vi "OpenExcel.vi"(1 "Visible(T)":bool=TRUE, 2 "error in (no error)":errorcluster caption="错误输入（无错误）", 4 "输入Excel路径":path) -> (0 "error out":errorcluster caption="错误输出")   [LabVIEW 2018]
panel:
  in  "Excel._Application":refnum<k7>
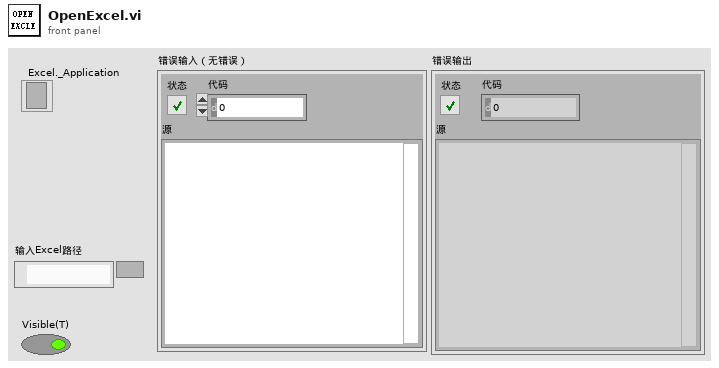
[diagram p1: front panel]
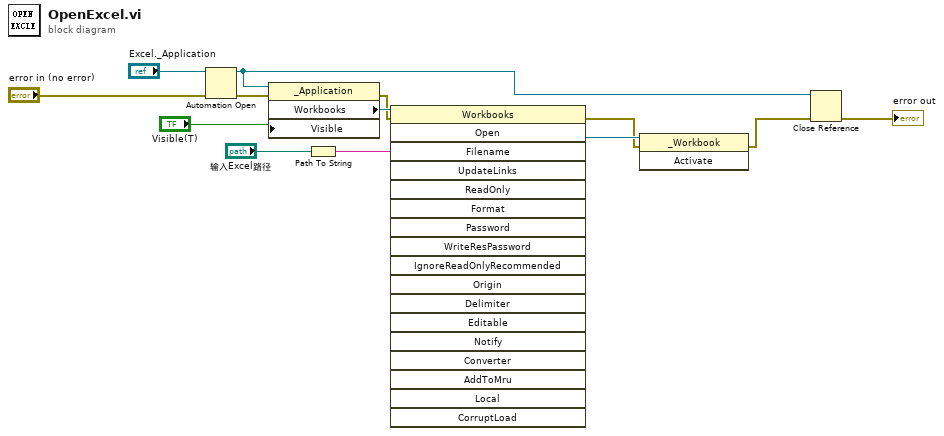
[diagram p0: block diagram]
diagram:
  n1 = Automation Open(error in (no error)="error in (no error)", Automation Refnum="Excel._Application") -> (Automation Refnum=w5:refnum<k7>, error out=w7:errorcluster)  [unwired: 2 in]
  n2 = property class="_Application"(reference=w5, error in=w7, "Visible"="Visible(T)") -> (error out=w10:errorcluster, "Workbooks"=w13:refnum<k7>)  [unwired: 1 out]
  n3 = Path To String(path="输入Excel路径") -> (string=w11:string)
  n4 = invoke on="调用节点" class="Workbooks" method="Open"(reference=w13, error in=w10, "Filename"=w11) -> (error out=w2:errorcluster, "Open"=w3:refnum<k7>)  [unwired: 15 in, 16 out]
  n5 = invoke class="_Workbook" method="Activate"(reference=w3, error in=w2) -> (error out=w1:errorcluster)  [unwired: 1 in, 2 out]
  n6 = Close Reference(reference=w5, error in (no error)=w1) -> (error out=→"error out":errorcluster)
